vi "UI(Edit_Channel_Init).vi"(11 "Cluster":T1) -> ()   [LabVIEW 2025, in "DAQ_Module.lvlib" / "DAQ_Module.lvclass"]
uses:
  DAQ_Module.lvclass
  DAQ_Module.lvclass/DAQ_Module.ctl
  4202103b-45c1-4860-a76d-89cab181edc9.vi
  DAQ_AI_Task_Config.ctl
  a2923e9f-e188-40ea-a9fb-ca3040fb7d44.vi
  DAQ_Linear_Task_Config.ctl
  7bc8e810-feac-4d08-b0fa-f77e1f4e2c83.vi
  DAQ_Angular_Task_Config.ctl
  DAQ_Task_Type.ctl
  DAQ_SampleRateConfig.ctl
  DAQ_HW_Type.ctl
  DAQ_Task_Config.ctl
  DAQ_Config.ctl
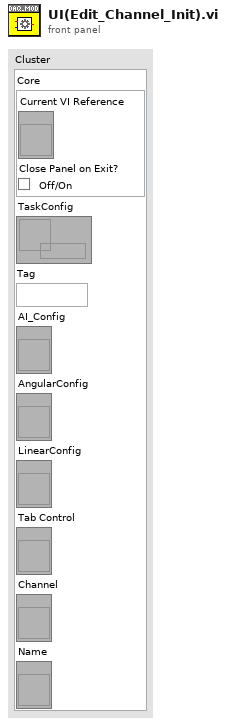
[diagram p1: front panel]
types:
  T1 = cluster{"Core":cluster{"Current VI Reference":refnum<vi>, "Close Panel on Exit?":bool}, "TaskConfig":refnum<data-value>, "Tag":string, "AI_Config":refnum<vi>, "AngularConfig":refnum<vi>, "LinearConfig":refnum<vi>, "Tab Control":refnum<vi>, "Channel":refnum<vi>, "Name":refnum<vi>}
  T2 = typedef "DAQ_Module.lvlib/DAQ_Module.lvclass/DAQ_AI_Task_Config.ctl" = cluster{"MaxValue":dbl, "MinValue":dbl, "InputTerminalConfiguration":i32}
  T3 = typedef "DAQ_Module.lvlib/DAQ_Module.lvclass/DAQ_Linear_Task_Config.ctl" = cluster{"decoding type":i32, "units":i32, "distance per pulse":dbl, "initial position":dbl, "z index enable":bool, "z index value":dbl, "z index phase":i32, "CI_Encoder_A_InputTerm":string, "CI_Encoder_B_InputTerm":string, "CI_Encoder_Z_InputTerm":string}
  T4 = typedef "DAQ_Module.lvlib/DAQ_Module.lvclass/DAQ_Angular_Task_Config.ctl" = cluster{"decoding type":i32, "units":i32, "pulses per revolution":u32, "initial angle":dbl, "z index enable":bool, "z index value":dbl, "z index phase":i32, "CI_Encoder_A_InputTerm":string, "CI_Encoder_B_InputTerm":string, "CI_Encoder_Z_InputTerm":string}
  T5 = typedef "DAQ_Module.lvlib/DAQ_Module.lvclass/DAQ_Config.ctl" = map{string, T6}
  T6 = typedef "DAQ_Module.lvlib/DAQ_Module.lvclass/DAQ_Task_Config.ctl" = cluster{"Drive":T7, "TaskType":T8, "PhysicalChannels":string, "SampleRateConfiguration":T9, "ChannelConfig":map{string, cluster{"Name":string, "Config":string}}, "Enable":bool, "ShowPanel":bool}
  T7 = typedef "DAQ_Module.lvlib/DAQ_Module.lvclass/DAQ_HW_Type.ctl" = enum16{"NI_DAQmx", "Simulated_DAQ"}
  T8 = typedef "DAQ_Module.lvlib/DAQ_Module.lvclass/DAQ_Task_Type.ctl" = enum16{"AI", "Linear", "Angular", "AO"}
  T9 = typedef "DAQ_Module.lvlib/DAQ_Module.lvclass/DAQ_SampleRateConfig.ctl" = cluster{"SampleRate":dbl, "SamplesPerChannel":u32, "SamplesPerRead":i32, "SampleMode":i32, "Clock Source":string}
  T10 = map{string, cluster{"Name":string, "Config":string}}
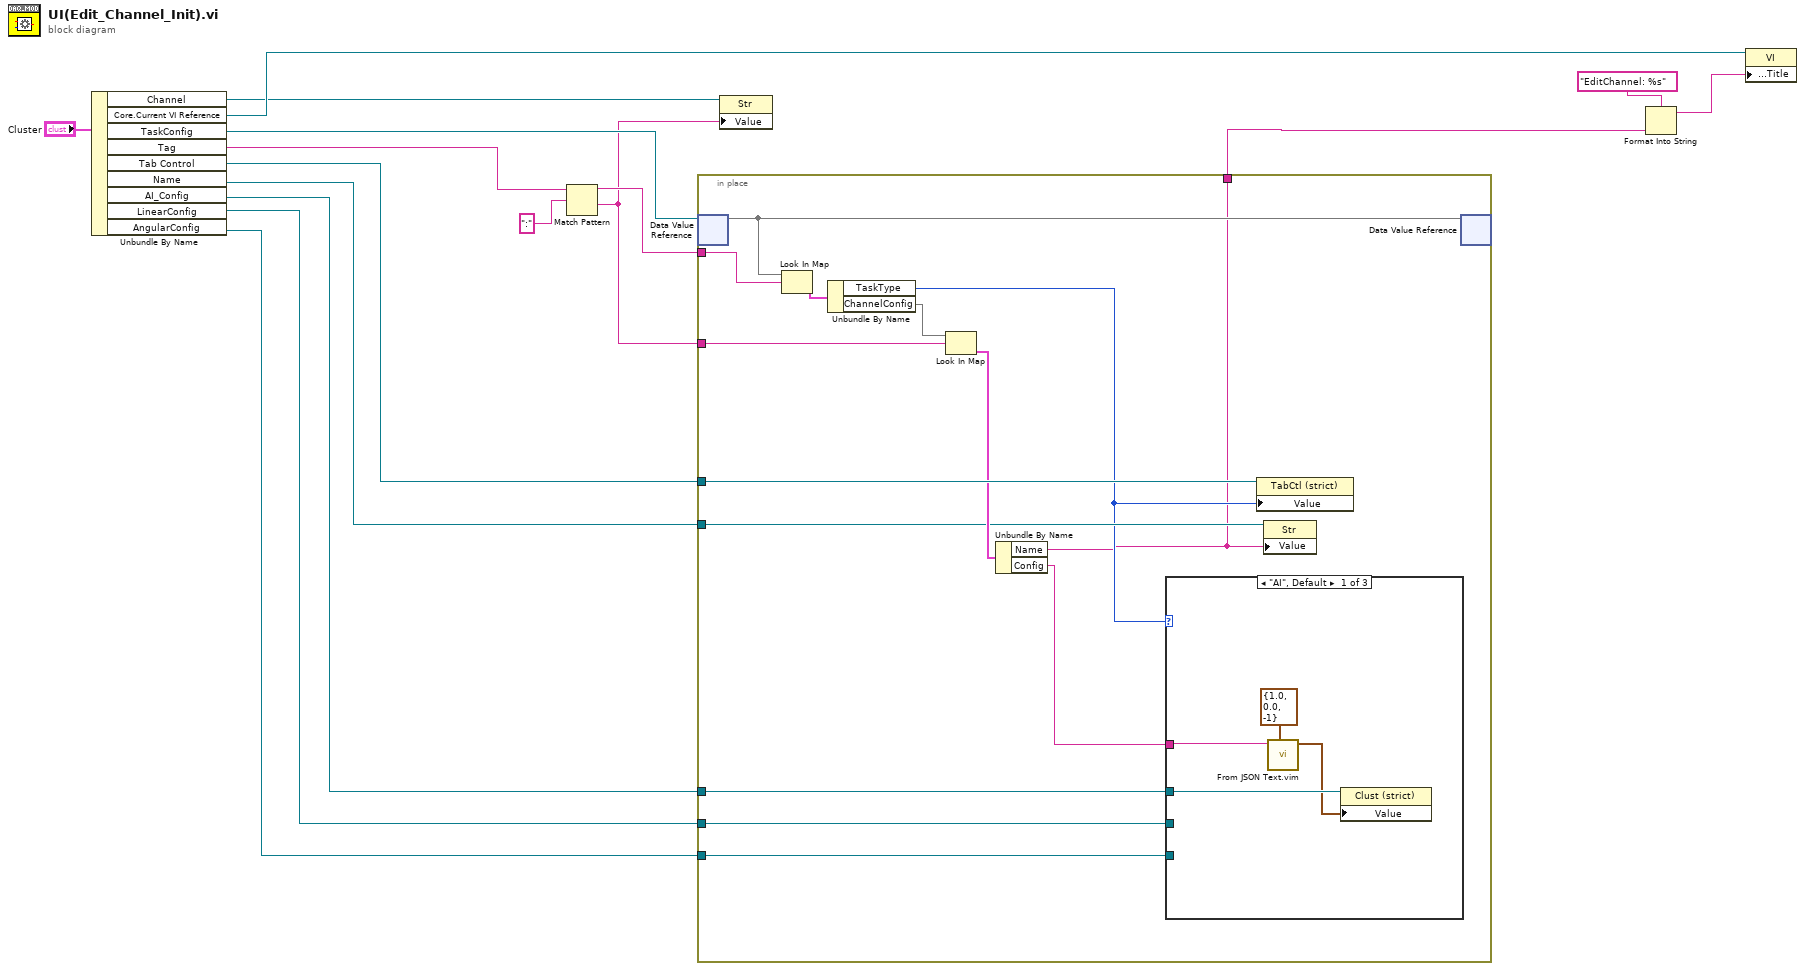
[diagram p0: block diagram]
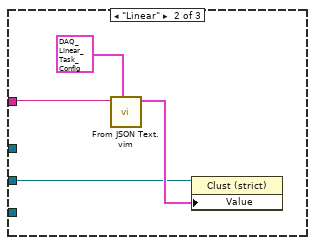
[diagram p2: hidden frame]
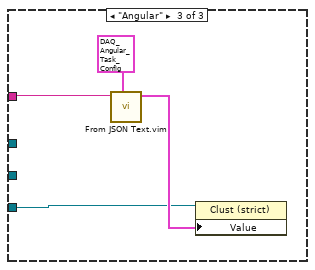
[diagram p3: hidden frame]
diagram:
  n1 = Unbundle By Name("Cluster") -> ("Channel"=w2:refnum<vi>, "Core.Current VI Reference"=w4:refnum<vi>, "TaskConfig"=w13:refnum<data-value>, "Tag"=w12:string, "Tab Control"=w11:refnum<vi>, "Name"=w10:refnum<vi>, "AI_Config"=w9:refnum<vi>, "LinearConfig"=w8:refnum<vi>, "AngularConfig"=w7:refnum<vi>)
  n2 = Match Pattern(string=w12, regular expression=":") -> (before substring=w15:string, after substring=w1:string)  [unwired: 1 in, 2 out]
  n3 = in-place {
    in-place-border: w15 -> [w29]
    in-place-border: w1 -> [w26]
    in-place-border: w11 -> [w25]
    in-place-border: w10 -> [w23]
    in-place-border: w9 -> [w20]
    in-place-border: w8 -> [w19]
    in-place-border: w7 -> [w18]
    in-place-border: [w17] -> w3
    n4 = in-place-dvr #1(w13) -> (w30:T5)  [unwired: 1 out]
    n5 = Look In Map(map=w30, key=w29) -> (value=w28:T6)  [unwired: 1 in, 1 out]
    n6 = Unbundle By Name(w28) -> ("TaskType"=w22:T8, "ChannelConfig"=w27:T10)
    n7 = Look In Map(map=w27, key=w26) -> (value=w24:cluster{"Name":string, "Config":string})  [unwired: 1 in, 1 out]
    n8 = Unbundle By Name(w24) -> ("Name"=w17:string, "Config"=w21:string)
    n9 = case shown="\"AI\", Default" w22 {
      tunnel: w21 -> [w34 w38 w42]
      tunnel: w20 -> [w32 _ _]
      tunnel: w19 -> [_ w35 _]
      tunnel: w18 -> [_ _ w39]
      frame "AI", Default {
        n10 = call "From JSON Text.vim"("Data Type and Default Value"=T2 {"MaxValue"=1.0, "MinValue"=0.0, "InputTerminalConfiguration"=-1} ("AI_Config"), "JSON"=w34) -> ("Data out"=w31:T2)  [unwired: 8 in, 1 out]
        n11 = property class="Clust (strict)"(reference=w32, "Value"=w31) -> ()  [unwired: 1 in, 2 out]
      }
      frame "Linear" {
        n12 = call "From JSON Text.vim"("Data Type and Default Value"=T3 {"decoding type"=10092, "units"=10219, "distance per pulse"=0.001, "initial position"=0.0, "z index enable"=FALSE, "z index value"=0.0, "z index phase"=10040, "CI_Encoder_A_InputTerm"="", "CI_Encoder_B_InputTerm"="", "CI_Encoder_Z_InputTerm"=""} ("LinearConfig"), "JSON"=w38) -> ("Data out"=w37:T3)  [unwired: 8 in, 1 out]
        n13 = property class="Clust (strict)"(reference=w35, "Value"=w37) -> ()  [unwired: 1 in, 2 out]
      }
      frame "Angular" {
        n14 = call "From JSON Text.vim"("Data Type and Default Value"=T4 {"decoding type"=10092, "units"=10146, "pulses per revolution"=24, "initial angle"=0.0, "z index enable"=FALSE, "z index value"=0.0, "z index phase"=10040, "CI_Encoder_A_InputTerm"="", "CI_Encoder_B_InputTerm"="", "CI_Encoder_Z_InputTerm"=""} ("AngularConfig"), "JSON"=w42) -> ("Data out"=w41:T4)  [unwired: 8 in, 1 out]
        n15 = property class="Clust (strict)"(reference=w39, "Value"=w41) -> ()  [unwired: 1 in, 2 out]
      }
    }
    n16 = property class="TabCtl (strict)"(reference=w25, "Value"=w22) -> ()  [unwired: 1 in, 2 out]
    n17 = property class="Str"(reference=w23, "Value"=w17) -> ()  [unwired: 1 in, 2 out]
    n18 = in-place-dvr #1(w30) -> ()  [unwired: 2 out]
  }
  n19 = property class="Str"(reference=w2, "Value"=w1) -> ()  [unwired: 1 in, 2 out]
  n20 = Format Into String(format string="EditChannel: %s", w3) -> (resulting string=w5:string)  [unwired: 2 in, 1 out]
  n21 = property class="VI"(reference=w4, "Front Panel.Title"=w5) -> ()  [unwired: 1 in, 2 out]
